vi "Read data.vi"(8 "error in":errorcluster, 9 "starting address":u16, 10 "number of inputs":u16, 11 "Modbus master in":refnum<class "Modbus Master.lvclass">) -> (0 "error out":errorcluster, 2 "register values":u16[](array[numeric]), 3 "Modbus master out":refnum<class "Modbus Master.lvclass">)   [LabVIEW 2023, in "RS485.lvlib"]
uses:
  RS485.lvlib
  <vilib>/NI/Modbus Library/API/Master/Modbus Master.lvclass
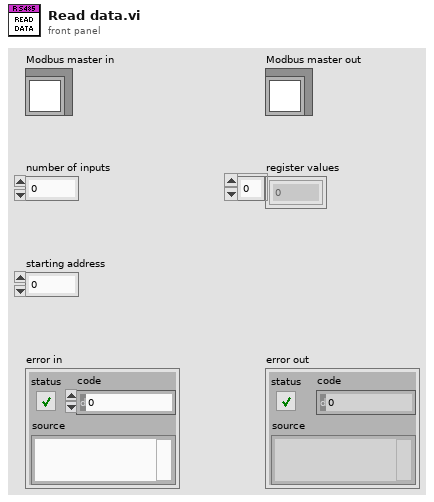
[diagram p1: front panel]
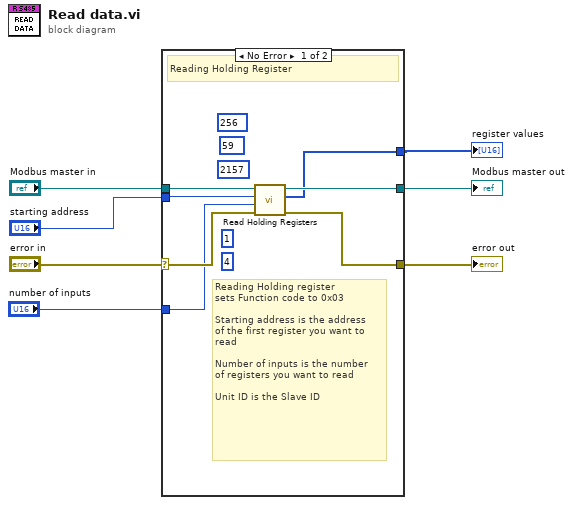
[diagram p0: block diagram]
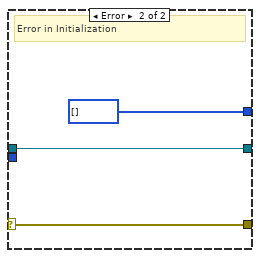
[diagram p2: hidden frame]
diagram:
  n1 = case shown="No Error" "error in" {
    selector: "error in" -> [w11 w16]
    tunnel: "Modbus master in" -> [w13 w17]
    tunnel: [w14 w17] -> w2
    tunnel: [w12 w16] -> w1
    tunnel: "starting address" -> [w10 _]
    tunnel: "number of inputs" -> [w9 _]
    tunnel: [w8 u16[] [] ("register values")] -> w3
    frame No Error {
      (unwired) u16 2157 ("starting address")
      (unwired) u16 59 ("starting address")
      (unwired) u16 1 ("number of inputs")
      (unwired) u16 4 ("number of inputs")
      (unwired) u16 256 ("starting address")
      # "Reading Holding register\nsets Function code to 0x03\n\nStarting address is the address\nof the first register you want to\nread\n\nNumber of inputs is the number\nof registers you want to read\n\nUnit ID is the Slave ID"
      # "Reading Holding Register"
      n2 = call-dynamic "Read Holding Registers.vi"("error in"=w11, "number of inputs"=w9, "starting address"=w10, "Modbus master in"=w13) -> ("error out"=w12:errorcluster, "register values"=w8:u16[], "Modbus master out"=w14:refnum<class "Modbus Master.lvclass">)  [unwired: 5 in]
    }
    frame Error {
      # "Error in Initialization"
    }
  }
  "register values" <- w3
  "Modbus master out" <- w2
  "error out" <- w1
